vi "WaveformComponent, Create Stimulus Pulse.vi"(5 "Recovery Phase":T1={"offset"=-0.25, "amplitude"=-2.0, "delay"=4.9999999999999996e-05, "leading edge"=2.4999999999999998e-05, "pulse width"=0.0003, "trailing edge"=9.999999999999999e-05, "ref level %"=33.3} {"ref level %" format="%.1f"; "offset" format="%.3f"; "pulse width" format="%.1f"; "trailing edge" format="%.1f"; "amplitude" format="%.3f"; "delay" format="%.1f"; "leading edge" format="%.1f"}, 6 "burst count (1)":i32=1 min=1 step=1, 7 "Stimulus Phase":T1={"offset"=0.25, "amplitude"=2.0, "delay"=0.00019999999999999998, "leading edge"=4.9999999999999996e-05, "pulse width"=0.00039999999999999996, "trailing edge"=4.9999999999999996e-05, "ref level %"=33.3} {"ref level %" format="%.1f"; "offset" format="%.3f"; "pulse width" format="%.1f"; "trailing edge" format="%.1f"; "amplitude" format="%.3f"; "delay" format="%.1f"; "leading edge" format="%.1f"}, 8 "error in":errorcluster, 9 "noise (0.1)":dbl[unit]=0.1 min=0.0 step=0.1 format="%.3f", 10 "frequency":dbl[unit]=330.0 format="%.1f", 11 "waveform in":waveform(dbl)={"t0"=timestamp(3474892848.0780005 s since 1904-01-01), "dt"=1e-06, "Y"=[]}) -> (0 "error out":errorcluster, 3 "waveform out":waveform(dbl)(graph)={"t0"=timestamp(3474892848.0780005 s since 1904-01-01), "dt"=1e-06, "Y"=[]})   [LabVIEW 2010]
uses:
  Pulse Parameters.ctl
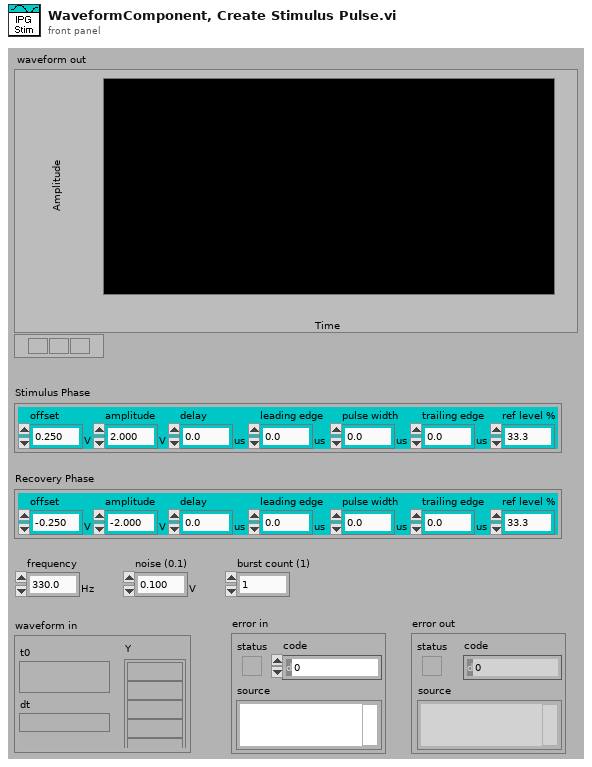
[diagram p1: front panel]
types:
  T1 = typedef "Pulse Parameters.ctl" = cluster{"offset":dbl[unit], "amplitude":dbl[unit], "delay":dbl[unit], "leading edge":dbl[unit], "pulse width":dbl[unit], "trailing edge":dbl[unit], "ref level %":dbl}
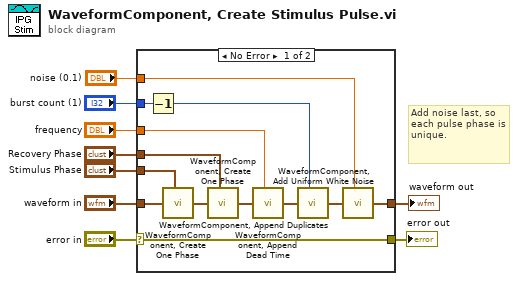
[diagram p0: block diagram]
diagram:
  # "Add noise last, so each pulse phase is unique."
  n1 = case shown="No Error" "error in" {
    selector: "error in" -> [w10 w24]
    tunnel: "waveform in" -> [w22 w23]
    tunnel: "Stimulus Phase" -> [w21 _]
    tunnel: "Recovery Phase" -> [w20 _]
    tunnel: "frequency" -> [w19 _]
    tunnel: "noise (0.1)" -> [w16 _]
    tunnel: "burst count (1)" -> [w15 _]
    tunnel: [w11 w23] -> w3
    tunnel: [w10 w24] -> w1
    frame No Error {
      n2 = Decrement(x=w15) -> (x-1=w14:i32)
      n3 = call "WaveformComponent, Create One Phase.vi"("waveform in"=w22, "phase parameters"=w21) -> ("waveform out"=w18:waveform(dbl))  [unwired: 1 in]
      n4 = call "WaveformComponent, Create One Phase.vi"("waveform in"=w18, "phase parameters"=w20) -> ("waveform out"=w17:waveform(dbl))  [unwired: 1 in]
      n5 = call "WaveformComponent, Append Dead Time.vi"("waveform in"=w17, "frequency"=w19) -> ("waveform out"=w13:waveform(dbl))  [unwired: 1 in]
      n6 = call "WaveformComponent, Append Duplicates.vi"("waveform"=w13, "duplicates"=w14) -> ("waveform out"=w12:waveform(dbl))  [unwired: 1 in]
      n7 = call "WaveformComponent, Add Uniform White Noise.vi"("waveform"=w12, "level (1.0)"=w16) -> ("waveform out"=w11:waveform(dbl))  [unwired: 1 in]
    }
    frame Error {
    }
  }
  "error out" <- w1
  "waveform out" <- w3
